vi "Compute Checksum_old.vi"(0 "Main time":u16, 5 "Group Time":u8, 7 "N factor":u8, 9 "Channel Stim":u8, 11 "Channel LF":u8) -> (4 "Checksum":u8)   [LabVIEW 2019]
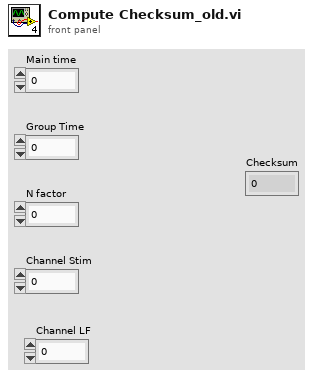
[diagram p1: front panel]
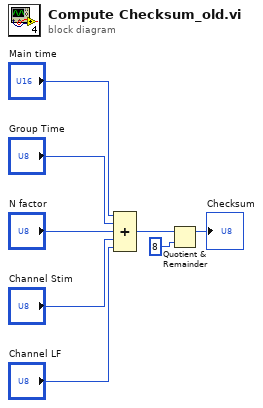
[diagram p0: block diagram]
diagram:
  n1 = Compound Arithmetic op=ADD("Main time", "Group Time", "N factor", "Channel Stim", "Channel LF") -> (w3:u16)
  n2 = Quotient & Remainder(x=w3, y=8) -> (x-y*floor(x/y)=→"Checksum":i32)  [unwired: 1 out]
